vi "PEM Query Wavelength.vi"(8 "error in (no error)":errorcluster, 11 "VISA resource name":refnum<visa-resource-name>="COM1") -> (0 "error out":errorcluster, 2 "Wavelength":dbl[unit], 3 "VISA resource name out":refnum<visa-resource-name>)   [LabVIEW 2017]
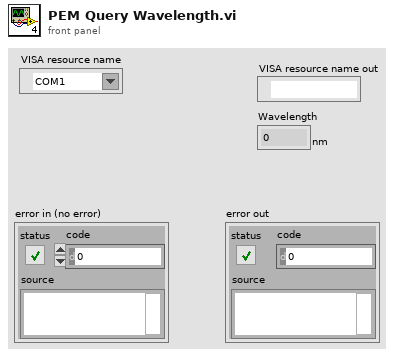
[diagram p1: front panel]
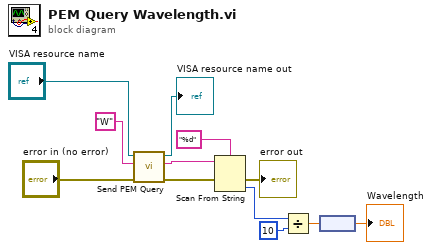
[diagram p0: block diagram]
diagram:
  n1 = call "Send PEM Query.vi"("error in (no error)"="error in (no error)", "query string"="W" ("write buffer"), "VISA resource name"="VISA resource name") -> ("error out"=w6:errorcluster, "query output"=w8:string, "VISA resource name out"=→"VISA resource name out":refnum<visa-resource-name>)  [unwired: 5 in, 1 out]
  n2 = Scan From String(format string="%d", input string=w8, error in=w6) -> (error out=→"error out":errorcluster, output 1=w4:i32)  [unwired: 2 in, 2 out]
  n3 = Divide(x=w4, y=10) -> (x/y=w2:dbl)
  n4 = node(w2) -> (→"Wavelength":dbl[unit])
